vi "反算.vi"(8 "error in (no error)":errorcluster caption="错误输入（无错误）", 10 "公式":cluster{"X^2":dbl, "X":dbl, "B":dbl}, 11 "监测值":dbl) -> (0 "error out":errorcluster caption="错误输出", 3 "信号值":dbl)   [LabVIEW 2016, in "斯坦道CODMn.lvlib"]
uses:
  <vilib>/Analysis/polynomials.llb/Polynomial Roots (DBL).vi
  <vilib>/Analysis/polynomials.llb/Polynomial Plot (Range).vi
  <vilib>/Analysis/NI_AALPro.lvlib
panel:
  out "Real Roots":dbl[](array[numeric]) caption="实数根"
  out "polynomial plot":cluster{dbl[], "P(A)":dbl[]}(graph) caption="多项式曲线"
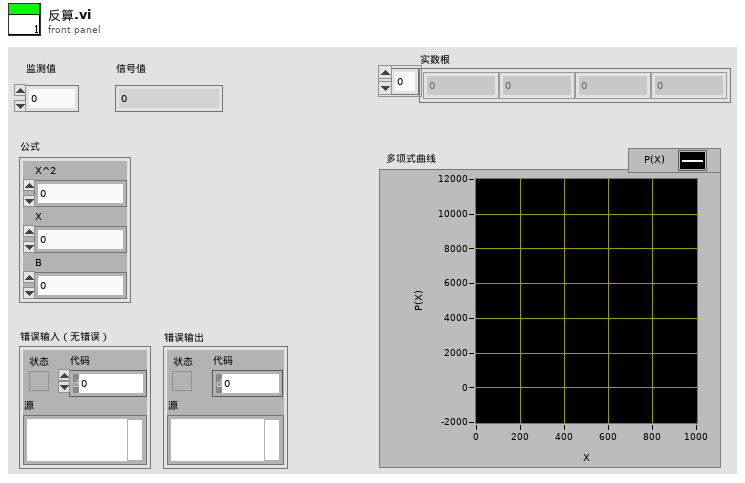
[diagram p1: front panel]
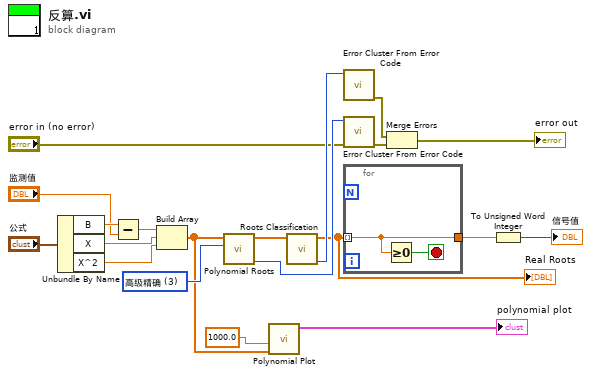
[diagram p0: block diagram]
diagram:
  w20 = u16 3 items=["常规", "简单分类", "精确", "高级精确"] ("option")
  n1 = Unbundle By Name("公式") -> ("B"=w18:dbl, "X"=w15:dbl, "X^2"=w14:dbl)
  n2 = Subtract(x=w18, y="监测值") -> (x-y=w16:dbl)
  n3 = Build Array(w16, w15, w14) -> (w12:dbl[])
  n4 = call-poly <vilib>:"Polynomial Roots.vi"("option"=w20, "P(x)"=w12) -> ("error"=w13:i32, "Roots"=w10:cdb[])  [unwired: 8 in]
  n5 = call-poly <vilib>:"Polynomial Plot.vi"("P(x)"=w12, "end"=1000.0) -> ("polynomial plot"=→"polynomial plot":cluster{"Ramp Pattern":dbl[], "P(A)":dbl[]})  [unwired: 8 in, 1 out]
  n6 = call <vilib>:"Roots Classification.vi"("Roots"=w10) -> ("error"=w8:i32, "Real Roots"=w4:dbl[])  [unwired: 7 in, 2 out]
  "Real Roots" <- w4
  n7 = call <vilib>:"Error Cluster From Error Code.vi"("error code (0)"=w8) -> ("error out"=w7:errorcluster)  [unwired: 8 in]
  n8 = call <vilib>:"Error Cluster From Error Code.vi"("error in (no error)"="error in (no error)", "error code (0)"=w13) -> ("error out"=w6:errorcluster)  [unwired: 7 in]
  n9 = for {
    tunnel: w4 -> [w22] mode=indexing
    tunnel: [w22] -> w2
    stop <- w21 stop-if-true
    n10 = Greater Or Equal To 0?(x=w22) -> (x >= 0?=w21:bool)
  }
  n11 = Merge Errors(w7, w6) -> (→"error out":errorcluster)
  n12 = To Unsigned Word Integer(number=w2) -> (unsigned 16bit integer=→"信号值":u16)
